vi "Receive Messages.vi"(8 "error in":errorcluster, 10 "Sender":string, 11 "PCAN-USB Read-Write Raw CAN Frame Strategy in":refnum<class "PCAN Read-Write Raw CAN Frame Strategy.lvclass">) -> (0 "error out":errorcluster, 2 "Messages":refnum<class "IMessage.lvclass">[](array[class]), 3 "PCAN-USB Read-Write Raw CAN Frame Strategy out":refnum<class "PCAN Read-Write Raw CAN Frame Strategy.lvclass">)   [LabVIEW 2024, in "PCAN Read-Write Raw CAN Frame Strategy.lvclass"]
uses:
  PCAN Read-Write Raw CAN Frame Strategy.lvclass
  PCAN Read-Write Raw CAN Frame Strategy.lvclass/PCAN Read-Write Raw CAN Frame Strategy.ctl
  Source/Messages/CAN Message/CAN Message.lvclass
  PCAN-USB Base Strategy/PCAN Base Strategy.lvclass
  Source/Interfaces/IMessage/IMessage.lvclass
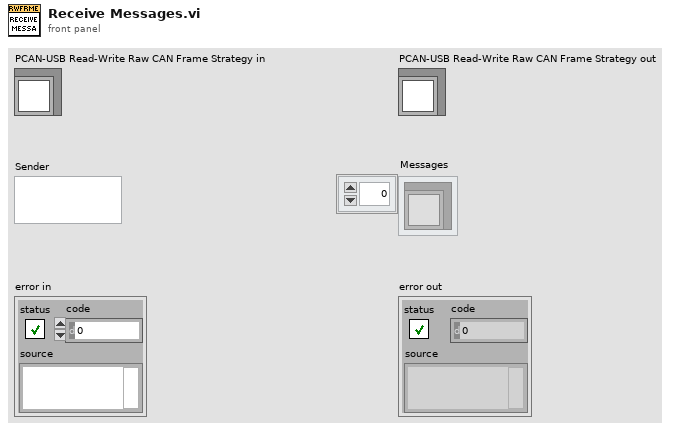
[diagram p1: front panel]
types:
  T1 = typedef "TPCANHandle.ctl" = enum16{"PCAN_NONEBUS  0x000", "PCAN_ISABUS1  0x21", "PCAN_ISABUS2  0x22", "PCAN_ISABUS3  0x23", "PCAN_ISABUS4  0x24", "PCAN_ISABUS5  0x25", "PCAN_ISABUS6  0x26", "PCAN_ISABUS7  0x27", "PCAN_ISABUS8  0x28", "PCAN_DNGBUS1  0x31", "PCAN_PCIBUS1  0x41", "PCAN_PCIBUS1  0x42", "PCAN_PCIBUS1  0x43", "PCAN_PCIBUS1  0x44", "PCAN_PCIBUS1  0x45", "PCAN_PCIBUS1  0x46", "PCAN_PCIBUS1  0x47", "PCAN_PCIBUS1  0x48", "PCAN_PCIBUS1  0x409", "PCAN_PCIBUS1  0x40A", "PCAN_PCIBUS1  0x40B", "PCAN_PCIBUS1  0x40C", "PCAN_PCIBUS1  0x40D", "PCAN_PCIBUS1  0x40E", "PCAN_PCIBUS1  0x40F", "PCAN_PCIBUS1  0x410", "PCAN_USBBUS1  0x51", "PCAN_USBBUS2  0x52", "PCAN_USBBUS3  0x53", "PCAN_USBBUS4  0x54", "PCAN_USBBUS5  0x55", "PCAN_USBBUS6  0x56", "PCAN_USBBUS7  0x57", "PCAN_USBBUS8  0x58", "PCAN_USBBUS9  0x509", "PCAN_USBBUS10  0x50A", "PCAN_USBBUS11  0x50B", "PCAN_USBBUS12  0x50C", "PCAN_USBBUS13  0x50D", "PCAN_USBBUS14  0x50E", "PCAN_USBBUS15  0x50F", "PCAN_USBBUS16  0x510", "PCAN_PCCBUS1  0x61", "PCAN_PCCBUS2  0x62", "PCAN_LANBUS1  0x801", "PCAN_LANBUS2  0x802", "PCAN_LANBUS3  0x803", "PCAN_LANBUS4  0x804", "PCAN_LANBUS5  0x805", "PCAN_LANBUS6  0x806", "PCAN_LANBUS7  0x807", "PCAN_LANBUS8  0x808", "PCAN_LANBUS9  0x809", "PCAN_LANBUS10  0x80A", "PCAN_LANBUS11  0x80B", "PCAN_LANBUS12  0x80C", "PCAN_LANBUS13  0x80D", "PCAN_LANBUS14  0x80E", "PCAN_LANBUS15  0x80F", "PCAN_LANBUS16  0x810"}
  T2 = typedef "TPCANTimestamp.ctl" = cluster{"millis overflow":u16, "millis ":u32, "micros":u16}
  T3 = typedef "CAN MSG Cluster.ctl" = cluster{"ID":u32, "MSG type":u8, "DLC":u8, "DATA":u8[]}
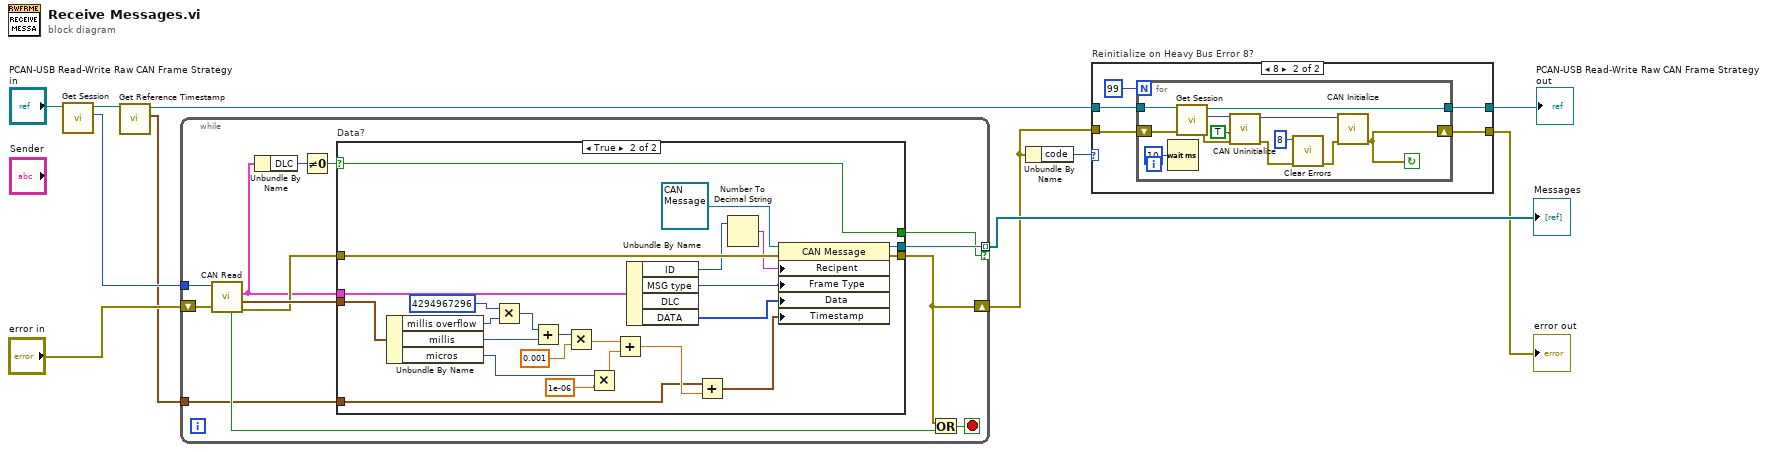
[diagram p0: block diagram]
diagram:
  n1 = call "Get Session.vi"("PCAN-USB Base Strategy in"="PCAN-USB Read-Write Raw CAN Frame Strategy in") -> ("TPCANHandle"=w10:T1, "PCAN-USB Base Strategy out"=w3:refnum<class "PCAN Read-Write Raw CAN Frame Strategy.lvclass">)  [unwired: 9 in]
  n2 = call "Get Reference Timestamp.vi"("PCAN Base Strategy in"=w3) -> ("Reference Timestamp"=w1:timestamp, "PCAN Base Strategy out"=w2:refnum<class "PCAN Read-Write Raw CAN Frame Strategy.lvclass">)  [unwired: 9 in]
  n3 = while {
    tunnel: w10 -> [w24]
    tunnel: [w21] -> w6 mode=indexing if=w13
    shift-right: [w18] -> w5
    shift-left: "error in" -> [w23]
    tunnel: w1 -> [w12]
    stop <- w19 stop-if-true
    n4 = call <instrlib>:"CAN Read.vi"("error in (no error)"=w23, "TPCANHandle"=w24) -> ("error out"=w20:errorcluster, "TPCANTimestamp out"=w22:T2, "CAN_Message out"=w16:T3, "rcv queue empty"=w17:bool)  [unwired: 5 in, 1 out]
    n5 = Unbundle By Name(w16) -> ("DLC"=w14:u8)
    n6 = Not Equal To 0?(x=w14) -> (x != 0?=w15:bool)
    n7 = case "Data?" shown="True" w15 {
      selector: w15 -> [w25 w34]
      tunnel: w22 -> [_ w50]
      tunnel: w16 -> [_ w49]
      tunnel: [_ w37] -> w21
      tunnel: w20 -> [w26 w36]
      tunnel: [w26 w35] -> w18
      tunnel: [w25 w34] -> w13
      tunnel: w12 -> [_ w27]
      frame False {
      }
      frame True {
        n8 = Unbundle By Name(w50) -> ("millis overflow"=w41:u16, "millis"=w44:u32, "micros"=w43:u16)
        n9 = Multiply(x=u64 4294967296, y=w41) -> (x*y=w39:u64)
        n10 = Add(x=w39, y=w44) -> (x+y=w40:u64)
        n11 = Multiply(x=w40, y=0.001) -> (x*y=w45:dbl)
        n12 = Multiply(x=w43, y=1e-06) -> (x*y=w46:dbl)
        n13 = Add(x=w45, y=w46) -> (x+y=w29:dbl)
        n14 = Unbundle By Name(w49) -> ("ID"=w33:u32, "MSG type"=w31:u8, "DATA"=w30:u8[])  [unwired: 1 out]
        n15 = Add(x=w27, y=w29) -> (x+y=w28:timestamp)
        n16 = Number To Decimal String(number=w33) -> (decimal integer string=w32:string)  [unwired: 1 in]
        n17 = property class="CAN Message"(reference=refnum<class "CAN Message.lvclass"> refnum ("CAN Message"), error in=w36, "Recipent"=w32, "Frame Type"=w31, "Data"=w30, "Timestamp"=w28) -> (reference out=w37:refnum<class "CAN Message.lvclass">, error out=w35:errorcluster)
      }
    }
    n18 = Or(x=w18, y=w17) -> (x .or. y?=w19:bool)
  }
  "Messages" <- w6
  n19 = Unbundle By Name(w5) -> ("code"=w8:i32)
  n20 = case "Reinitialize on Heavy Bus Error 8?" shown="8" w8 {
    tunnel: [w52 w57] -> w4
    tunnel: w5 -> [w52 w53]
    tunnel: w2 -> [w51 w56]
    tunnel: [w51 w55] -> w7
    frame Default {
    }
    frame 8 {
      n21 = for {
        N: 99 -> [_]
        shift-right: [w58] -> w57
        shift-left: w53 -> [w63]
        tunnel: w56 -> [w66]
        tunnel: [w65] -> w55
        stop <- w58 continue-if-true
        n22 = Wait (ms)(milliseconds to wait=u32 10) -> ()  [unwired: 1 out]
        n23 = call "Get Session.vi"("PCAN-USB Base Strategy in"=w66) -> ("TPCANHandle"=w64:T1, "PCAN-USB Base Strategy out"=w65:refnum<class "PCAN Read-Write Raw CAN Frame Strategy.lvclass">)  [unwired: 9 in]
        n24 = call <instrlib>:"CAN Uninitialize.vi"("error in (no error)"=w63, "Ignore input error"=TRUE, "TPCANHandle"=w64) -> ("error out"=w60:errorcluster, "TPCANHandle out"=w67:T1)  [unwired: 6 in, 1 out]
        n25 = call <vilib>:"Clear Errors.vi"("error in (no error)"=w60, "specific error code to clear (0: all)"=8) -> ("error out"=w59:errorcluster)  [unwired: 4 in, 1 out]
        n26 = call <instrlib>:"CAN Initialize.vi"("error in (no error)"=w59, "TPCANHandle"=w67) -> ("error out"=w58:errorcluster)  [unwired: 7 in, 2 out]
      }
    }
  }
  "error out" <- w4
  "PCAN-USB Read-Write Raw CAN Frame Strategy out" <- w7
